vi "TimingTest_withsynched.vi"() -> ()   [LabVIEW 2017]
uses:
  9d5949f9-07ca-45c6-940a-2e3a62ca42df.vi
  <vilib>/express/express analysis/Spectral/Block/exnSpectralBlock spectral measurements RMS poly.vi
  <vilib>/express/express analysis/Spectral/Block/exnSpectralBlock spectral measurements RMS array WFM.vi
  <vilib>/express/express analysis/Spectral/XNode/ExpressSpectralMeasurementsBlockNode.xnode
panel:
  in  "Samples to Read":i32=1000
  in  "Analog Input Sample Clock Source":tag="/Dev1/ao/SampleClock"
  out "Actual Update Generation Rate":dbl=5000.0 format="%0.2f"
  out "Actual Input Rate":dbl=10000.0 format="%0.2f"
  in  "rate":dbl=5000.0 caption="Update Generation Rate" format="%0.2f"
  in  "minimum value":dbl=-10.0 caption="Output Minimum Value" format="%0.2f"
  in  "maximum value":dbl=10.0 caption="Output Maximum Value" format="%0.2f"
  in  "physical channels":tag="Dev1/ao0" caption="Output Physical Channels"
  in  "Maximum Value":dbl=10.0 caption="Input Maximum Value" format="%0.2f"
  in  "Minimum Value":dbl=-10.0 caption="Input Minimum Value" format="%0.2f"
  in  "Rate":dbl=10000.0 caption="Input Rate" format="%0.2f"
  in  "Physical Channel":tag="Dev1/ai0" caption="Input Physical Channel"
  in  "100 Hz high-pass":bool
  out "Waveform Graph 2":cluster{"f0":dbl, "df":dbl, "magnitude":dbl[]}[](graph)
  out "Waveform Graph":waveform(dbl)[](graph)
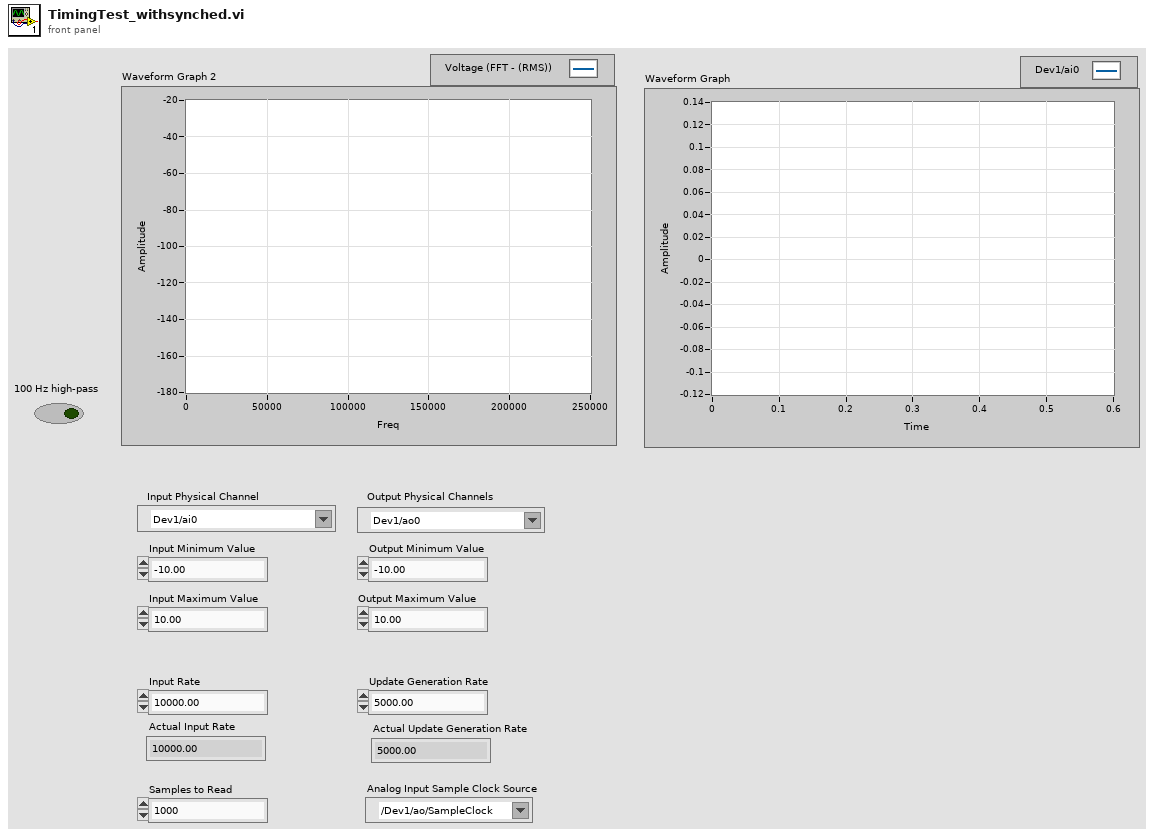
[diagram p1: front panel]
types:
  T1 = cluster{"averaging mode":u16, "weighting mode":u16, "number of averages":u32}
  T2 = cluster{"dB On (F)":bool, "unwrap phase (F)":bool, "convert to degree (F)":bool}
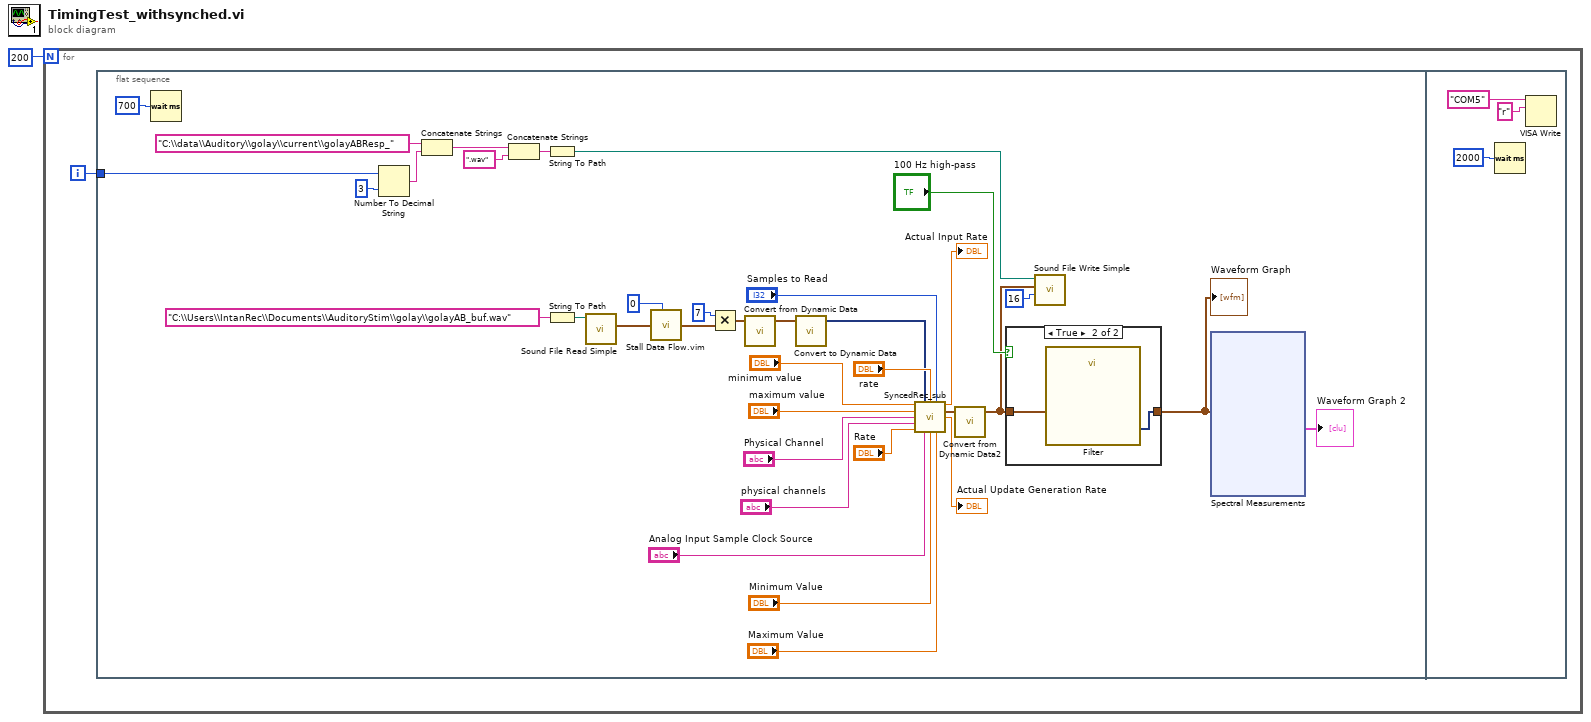
[diagram p0: block diagram]
diagram:
  n1 = for {
    N: 200 -> [_]
    i -> [w2]
    n2 = flat-sequence {
      tunnel: w2 -> [w34]
      frame #0 {
        n3 = Wait (ms)(milliseconds to wait=700) -> ()  [unwired: 1 out]
        n4 = Number To Decimal String(number=w34, width (-)=3) -> (decimal integer string=w32:string)
        n5 = Concatenate Strings("C:\\data\\Auditory\\golay\\current\\golayABResp_", w32) -> (w31:string)
        n6 = Concatenate Strings(w31, ".wav") -> (w29:string)
        n7 = String To Path(string=w29) -> (path=w36:path)
        n8 = String To Path(string="C:\\Users\\IntanRec\\Documents\\AuditoryStim\\golay\\golayAB_buf.wav") -> (path=w28:path)
        n9 = call <vilib>:"Sound File Read Simple.vi"("path"=w28) -> ("data"=w25:waveform(dbl)[])  [unwired: 7 in, 3 out]
        n10 = call "Stall Data Flow.vim"("value in"=w25, "milliseconds to wait"=0) -> ("value out"=w21:waveform(dbl)[])  [unwired: 1 out]
        n11 = Multiply(x=7, y=w21) -> (x*y=w6:waveform(dbl)[])
        n12 = call "Convert from Dynamic Data"("Dynamic Data Type"=w6) -> ("Waveform"=w5:waveform(dbl))  [unwired: 3 in]
        n13 = call "Convert to Dynamic Data"("Waveform"=w5) -> ("Dynamic Data Type"=w7:dynamicdata)  [unwired: 3 in]
        n14 = call "SyncedRec_sub.vi"("minimum value"="minimum value", "signal in"=w7, "rate"="rate", "Samples to Read"="Samples to Read", "maximum value"="maximum value", "Physical Channel"="Physical Channel", "physical channels"="physical channels", "Rate"="Rate", "Analog Input Sample Clock Source"="Analog Input Sample Clock Source", "Minimum Value"="Minimum Value", "Maximum Value"="Maximum Value") -> ("Actual Input Rate"=→"Actual Input Rate":dbl, "data"=w4:waveform(dbl), "Actual Update Generation Rate"=→"Actual Update Generation Rate":dbl)  [unwired: 2 in]
        n15 = call "Convert from Dynamic Data2"("Dynamic Data Type"=w4) -> ("Array of Waveform"=w3:waveform(dbl)[])  [unwired: 3 in]
        n16 = case shown="True" "100 Hz high-pass" {
          tunnel: w3 -> [w39 w41]
          tunnel: [w39 w40] -> w23
          frame False {
          }
          frame True {
            n17 = call "Filter"("Signal"=w41) -> ("Filtered Signal"=w40:dynamicdata)  [unwired: 9 in, 1 out]
          }
        }
        "Waveform Graph" <- w23
        n18 = call <vilib>:"Sound File Write Simple.vi"("bits per sample"=16, "data"=w3, "path"=w36) -> ()  [unwired: 7 in, 2 out]
        n19 = xnode "Spectral Measurements"("Signals"=w23) -> ("FFT - (RMS)"=→"Waveform Graph 2":cluster{"f0":dbl, "df":dbl, "magnitude":dbl[]}[])  [unwired: 1 in, 2 out]
      }
      frame #1 {
        n20 = Wait (ms)(milliseconds to wait=2000) -> ()  [unwired: 1 out]
        n21 = VISA Write(VISA resource name="COM5", write buffer="r") -> ()  [unwired: 1 in, 3 out]
      }
    }
  }
